vi "Get Named Attribute Value.vi"(8 "error in":errorcluster, 10 "Attribute Name":string, 11 "Node In":refnum<k20>) -> (0 "error out":errorcluster, 2 "Attribute Node":refnum<k20>, 3 "Node Out":refnum<k20>, 4 "Attribute Value":string)   [LabVIEW 2026]
uses:
  <resource>/objmgr/DOMUserDefRef.rc
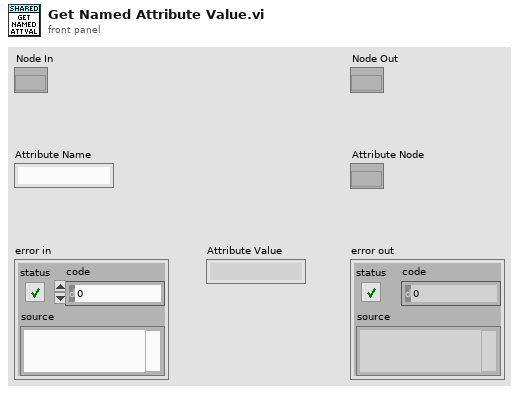
[diagram p1: front panel]
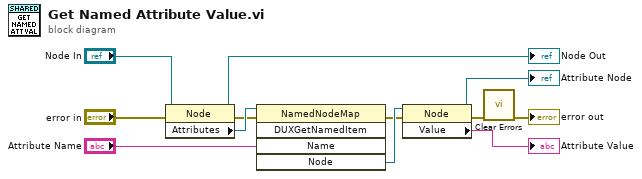
[diagram p0: block diagram]
diagram:
  n1 = property class="Node"(reference="Node In", error in="error in") -> (reference out=→"Node Out":refnum<k20>, error out=w5:errorcluster, "Attributes"=w6:refnum<k20>)
  n2 = invoke class="NamedNodeMap" method="DUXGetNamedItem"(reference=w6, error in=w5, "Name"="Attribute Name") -> (error out=w8:errorcluster, "Node"=w9:refnum<k20>)  [unwired: 2 in, 3 out]
  n3 = property class="Node"(reference=w9, error in=w8) -> (reference out=→"Attribute Node":refnum<k20>, error out=w11:errorcluster, "Value"=→"Attribute Value":string)
  n4 = call <vilib>:"Clear Errors.vi"("error in (no error)"=w11) -> ("error out"=→"error out":errorcluster)  [unwired: 5 in, 1 out]
